vi "Main.vi"() -> ()   [LabVIEW 2020]
uses:
  Definitions/Test States.ctl
  Definitions/State Types.ctl
  lv_src/Nominal Client/Nominal Client.lvclass
  lv_src/datasources/dataset/dataset.lvclass
  lv_src/Run/Run.lvclass
  lv_src/Nominal Client/Nominal Client.lvclass/Nominal Client.ctl
  48055549-f21b-4638-95ef-231369349838.vi
  <vilib>/Analysis/1siggen.llb/Ramp Pattern by Samples.vi
  <vilib>/DAQmx/write.llb/DAQmx Write (Analog DBL 1Chan 1Samp).vi
  dc8b2421-dc48-4948-9209-d90b052b0a2b.vi
  <extravilib>/ChannelInstances/Tag-bool/Write With Abort.vi
  lv_src/Nominal Client/private_data.set.vi
  <vilib>/Utility/file.llb/Application Directory.vi
  <vilib>/Utility/error.llb/Error Cluster From Error Code.vi
  submodules/reqwest-labview/lv-src/reqwest/create.vi
  lv_src/Nominal Client/Palette Items/who_am_i.vi
  lv_src/Nominal Client/asset.get.vi
  <vilib>/DAQmx/miscellaneous.llb/DAQmx Fill In Error Info.vi
  <extravilib>/ChannelInstances/Tag-bool/Instantiate.vi
  <extravilib>/ChannelInstances/Tag-bool/Endpoint.vi
  lv_src/User/User.lvclass
  lv_src/nominal types/workspace/workspace.lvclass
  submodules/reqwest-labview/lv-src/reqwest/reqwest.lvclass
  <vilib>/Analysis/NI_AALBase.lvlib
  lv_src/event/event.lvclass
  lv_src/asset/asset.lvclass
  submodules/nominal-streaming-labview-ffi/lv_src/Stream/Stream.lvclass
  <extravilib>/ChannelInstances/Tag-bool.lvlib
panel:
  out "Status":string
  out "Acceleration":waveform(dbl)[](graph)=[{"t0"=timestamp(3854950321.550671 s since 1904-01-01), "dt"=1.9999999999999998e-05, "Y"=array[50000 elements], "attributes"=variant("NI_ChannelName"=variant(string "Accelerometers/ai0"), "NI_UnitDescription"=variant(string "Volts"))}, {"t0"=timestamp(3854950321.550671 s since 1904-01-01), "dt"=1.9999999999999998e-05, "Y"=array[50000 elements], "attributes"=variant("NI_ChannelName"=variant(string "Accelerometers/ai1"), "NI_UnitDescription"=variant(string "Volts"))}, {"t0"=timestamp(3854950321.550671 s since 1904-01-01), "dt"=1.9999999999999998e-05, "Y"=array[50000 elements], "attributes"=variant("NI_ChannelName"=variant(string "VoltageInput/ai2"), "NI_UnitDescription"=variant(string "Volts"))}]
  out "Fan Speed":dbl[](graph)=[2691.1676625669315]
  out "Temperature":dbl(slide) scale=15.0..35.0
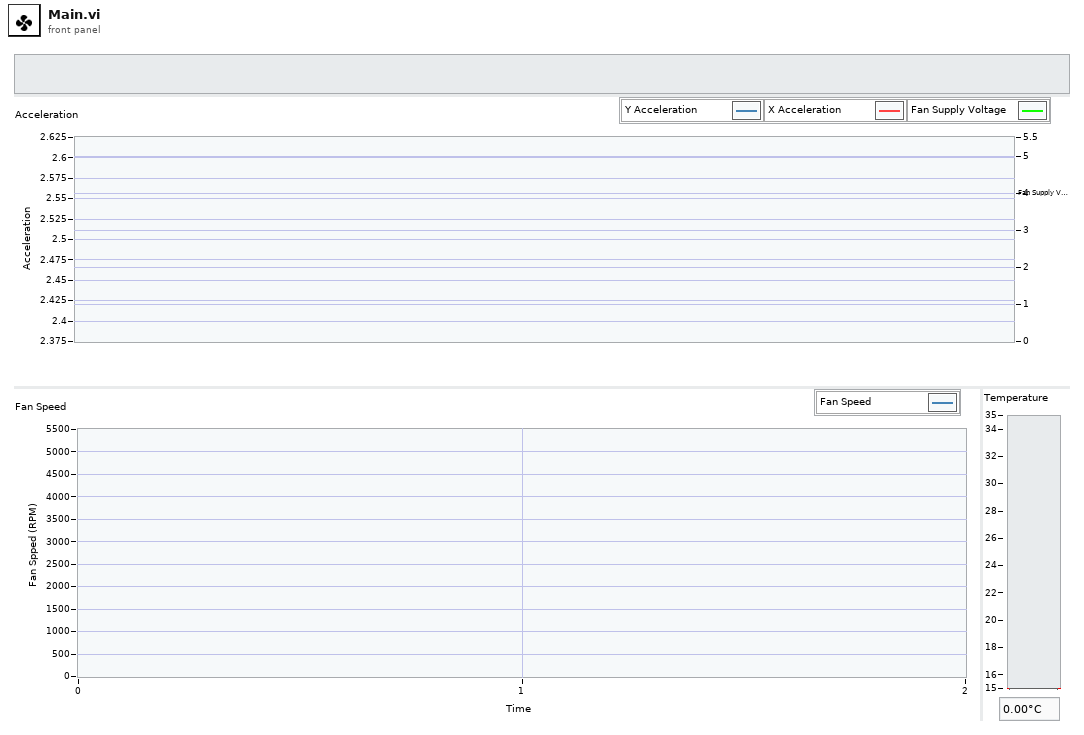
[diagram p1: front panel]
types:
  T1 = typedef "State Types.ctl" = cluster{"Nominal Client":refnum<class "Nominal Client.lvclass">, "dataset":refnum<class "dataset.lvclass">, "Run":refnum<class "Run.lvclass">, "Test Levels":dbl[], "Current Test Level":dbl, "DAQmx Task":refnum<k21>}
  T2 = typedef "Test States.ctl" = enum16{"Configuring Test Levels", "Setting Fan Voltage", "Fan Settling", "Test in Progress", "Setting Safe State", "Cooling Down"}
  T3 = typedef "Tag-bool.lvlib/))Channel.ctl" = refnum<queue>
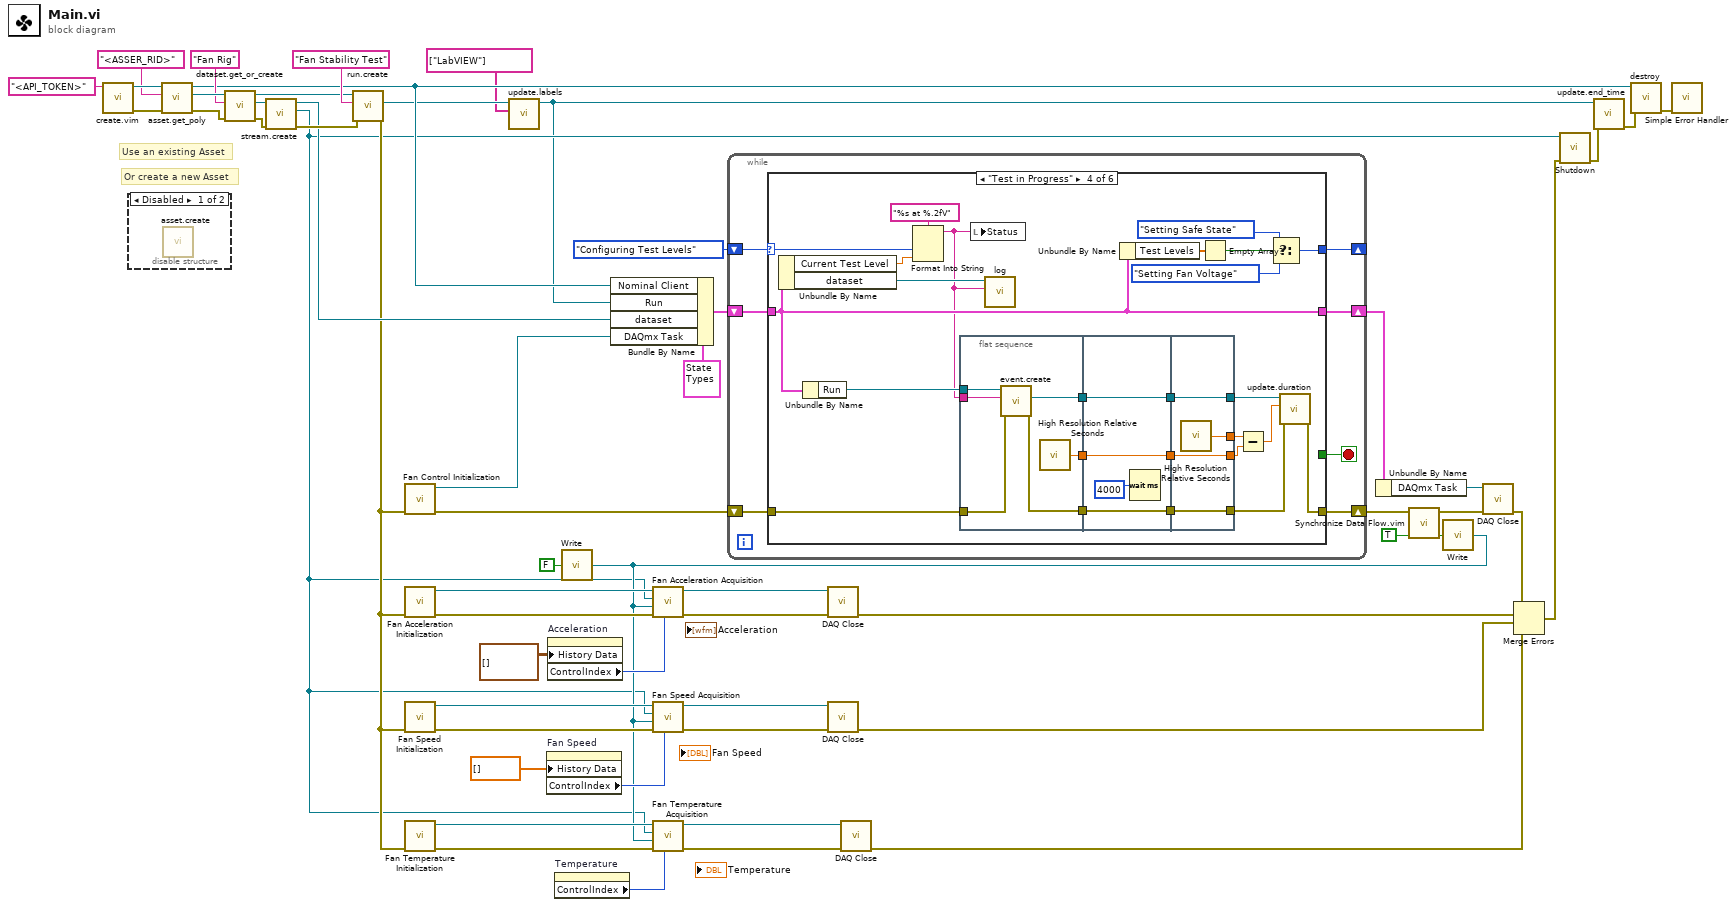
[diagram p0: block diagram]
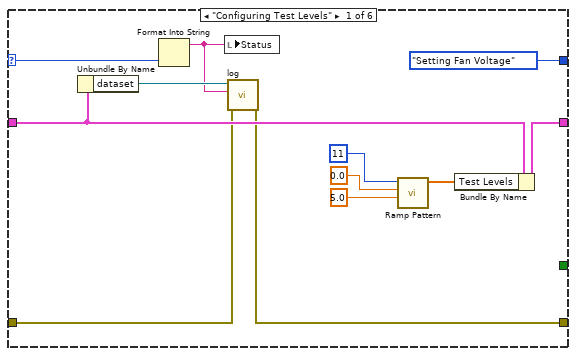
[diagram p3: hidden frame]
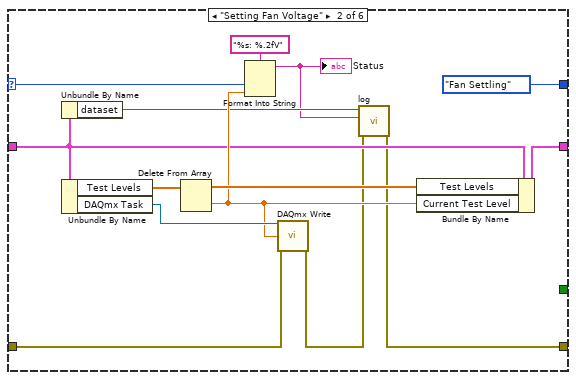
[diagram p4: hidden frame]
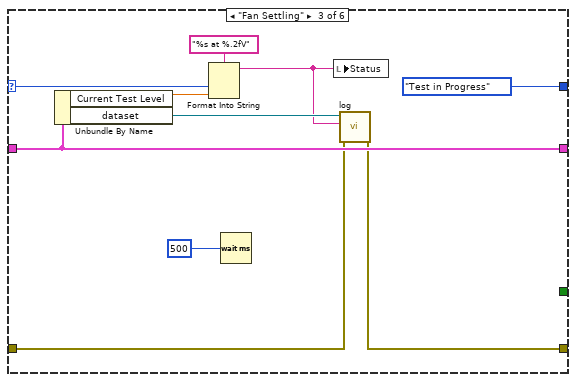
[diagram p5: hidden frame]
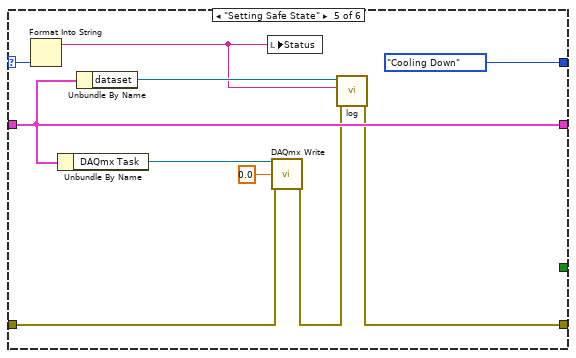
[diagram p6: hidden frame]
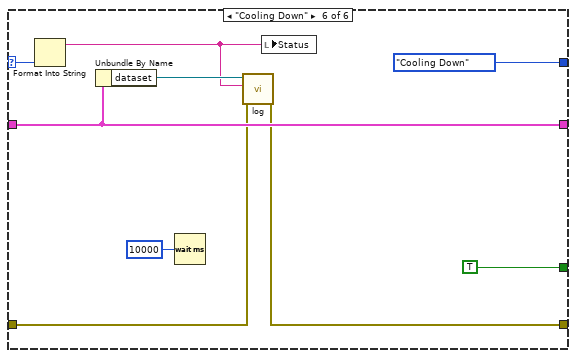
[diagram p7: hidden frame]
diagram:
  # "Or create a new Asset"
  # "Use an existing Asset"
  n1 = call "create.vim"("API Token (string or path)"="<API_TOKEN>") -> ("error out"=w55:errorcluster, "Nominal Client"=w57:refnum<class "Nominal Client.lvclass">)  [unwired: 8 in, 1 out]
  n2 = disable-structure shown="Disabled" {
    frame Disabled {
      n3 = call "asset.create.vi"() -> ()  [unwired: 9 in, 3 out]
    }
    frame Enabled {
    }
  }
  n4 = call-poly "asset.get_poly.vi"("error in"=w55, "Asset RID"="<ASSER_RID>", "Nominal Client in"=w57) -> ("error out"=w46:errorcluster, "Asset"=w52:refnum<class "asset.lvclass">, "Nominal Client out"=w39:refnum<class "Nominal Client.lvclass">)  [unwired: 6 in]
  n5 = call "dataset.get_or_create.vi"("error in"=w46, "Datascope Name"="Fan Rig", "asset in"=w52) -> ("error out"=w45:errorcluster, "dataset"=w50:refnum<class "dataset.lvclass">, "asset out"=w47:refnum<class "asset.lvclass">)  [unwired: 6 in]
  n6 = call "stream.create.vi"("error in (no error)"=w45, "dataset in"=w50) -> ("error out"=w44:errorcluster, "Stream"=w6:refnum<class "Stream.lvclass">, "dataset out"=w38:refnum<class "dataset.lvclass">)  [unwired: 7 in]
  n7 = call "run.create.vi"("error in"=w44, "Title"="Fan Stability Test", "asset in"=w47) -> ("error out"=w8:errorcluster, "Run"=w3:refnum<class "Run.lvclass">)  [unwired: 6 in, 1 out]
  n8 = call "Fan Control Initialization.vi"("error in"=w8) -> ("error out"=w13:errorcluster, "DAQmx Task"=w14:refnum<k21>)  [unwired: 9 in]
  n9 = call "Fan Acceleration Initialization.vi"("error in"=w8) -> ("error out"=w26:errorcluster, "DAQmx Task"=w27:refnum<k21>)  [unwired: 9 in]
  n10 = call "Fan Speed Initialization.vi"("error in"=w8) -> ("error out"=w24:errorcluster, "DAQmx Task Out"=w25:refnum<k21>)  [unwired: 9 in]
  n11 = call "Fan Temperature Initialization.vi"("error in"=w8) -> ("error out"=w11:errorcluster, "DAQmx Task"=w12:refnum<k21>)  [unwired: 9 in]
  n12 = call "update.labels.vi"("labels"=string[] ["LabVIEW"], "Run in"=w3) -> ("Run out"=w2:refnum<class "Run.lvclass">)  [unwired: 8 in, 1 out]
  n13 = property on="Fan Speed" class="WFChart (strict)"("History Data"=dbl[] []) -> ("ControlIndex"=w28:i32)  [unwired: 2 in, 2 out]
  n14 = property on="Acceleration" class="WFChart (strict)"("History Data"=waveform(dbl)[][] []) -> ("ControlIndex"=w29:i32)  [unwired: 2 in, 2 out]
  n15 = property on="Temperature" class="Slide (strict)"() -> ("ControlIndex"=w5:i32)  [unwired: 2 in, 2 out]
  n16 = call <extravilib>:"Write.vi"("element"=FALSE ("stop")) -> ("channel"=w7:T3)  [unwired: 1 out]
  n17 = Bundle By Name(cluster=T1 {"Nominal Client"=refnum, "dataset"=refnum, "Run"=refnum, "Test Levels"=[], "Current Test Level"=0.0, "DAQmx Task"=""} ("State Type"), "Nominal Client"=w39, "Run"=w2, "dataset"=w38, "DAQmx Task"=w14) -> (w37:T1)
  n18 = call "Fan Acceleration Acquisition.vi"("Acceleration Control Index"=w29, "error in"=w26, "stop"=w7, "Stream"=w6, "DAQmx Task In"=w27) -> ("error out"=w19:errorcluster, "DAQmx Task Out"=w20:refnum<k21>)  [unwired: 5 in]
  n19 = call "Fan Speed Acquisition.vi"("Control Index"=w28, "error in (no error)"=w24, "channel"=w7, "Stream in"=w6, "DAQmx Task In"=w25) -> ("error out"=w17:errorcluster, "DAQmx Task Out"=w18:refnum<k21>)  [unwired: 5 in]
  n20 = call "Fan Temperature Acquisition.vi"("Control Index"=w5, "error in (no error)"=w11, "channel"=w7, "Stream in"=w6, "DAQmx Task In"=w12) -> ("error out"=w10:errorcluster, "DAQmx Task Out"=w9:refnum<k21>)  [unwired: 5 in]
  n21 = while {
    shift-right: [w63] -> _
    shift-left: Test_States."Configuring Test Levels" ("states") -> [w64]
    shift-right: [w60] -> w35
    shift-left: w13 -> [w61]
    shift-right: [w58] -> w36
    shift-left: w37 -> [w59]
    stop <- w62 stop-if-true
    n22 = case shown="\"Test in Progress\"" w64 {
      selector: w64 -> [w72 w87 w98 w107 w146 w155]
      tunnel: [Test_States."Setting Fan Voltage" ("states") Test_States."Fan Settling" ("states") Test_States."Test in Progress" ("states") w122 Test_States."Cooling Down" ("states") Test_States."Cooling Down" ("states")] -> w63
      tunnel: [_ _ _ _ _ TRUE] -> w62
      tunnel: w61 -> [w66 w89 w93 w121 w147 w151]
      tunnel: [w65 w77 w92 w110 w140 w150] -> w60
      tunnel: w59 -> [w69 w81 w96 w104 w144 w154]
      tunnel: [w71 w85 w96 w104 w144 w154] -> w58
      frame "Configuring Test Levels" {
        n23 = Unbundle By Name(w69) -> ("dataset"=w68:refnum<class "dataset.lvclass">)
        n24 = Format Into String(w72) -> (resulting string=w67:string)  [unwired: 3 in, 1 out]
        n25 = local write "Status"(w67) -> ()
        n26 = call "log.vi"("error in (no error)"=w66, "Message"=w67, "dataset in"=w68) -> ("error out"=w65:errorcluster)  [unwired: 7 in, 1 out]
        n27 = call-poly <vilib>:"Ramp Pattern.vi"("start"=5.0 ("end"), "end"=0.0 ("start"), "samples"=11) -> ("Ramp Pattern"=w70:dbl[])  [unwired: 7 in, 1 out]
        n28 = Bundle By Name(cluster=w69, "Test Levels"=w70) -> (w71:T1)
      }
      frame "Setting Fan Voltage" {
        n29 = Unbundle By Name(w81) -> ("dataset"=w80:refnum<class "dataset.lvclass">)
        n30 = Unbundle By Name(w81) -> ("Test Levels"=w86:dbl[], "DAQmx Task"=w83:refnum<k21>)
        n31 = Delete From Array(array=w86) -> (deleted portion=w82:dbl, array with subset deleted=w84:dbl[])  [unwired: 2 in]
        n32 = Format Into String(format string="%s: %.2fV", w87, w82) -> (resulting string=w79:string)  [unwired: 2 in, 1 out]
        "Status" <- w79
        n33 = call-poly <vilib>:"DAQmx Write.vi"("task/channels in"=w83, "data"=w82, "error in"=w89) -> ("error out"=w78:errorcluster)  [unwired: 10 in, 2 out]
        n34 = call "log.vi"("error in (no error)"=w78, "Message"=w79, "dataset in"=w80) -> ("error out"=w77:errorcluster)  [unwired: 7 in, 1 out]
        n35 = Bundle By Name(cluster=w81, "Test Levels"=w84, "Current Test Level"=w82) -> (w85:T1)
      }
      frame "Fan Settling" {
        n36 = Unbundle By Name(w96) -> ("Current Test Level"=w95:dbl, "dataset"=w94:refnum<class "dataset.lvclass">)
        n37 = Format Into String(format string="%s at %.2fV", w98, w95) -> (resulting string=w91:string)  [unwired: 2 in, 1 out]
        n38 = Wait (ms)(milliseconds to wait=u32 500) -> ()  [unwired: 1 out]
        n39 = local write "Status"(w91) -> ()
        n40 = call "log.vi"("error in (no error)"=w93, "Message"=w91, "dataset in"=w94) -> ("error out"=w92:errorcluster)  [unwired: 7 in, 1 out]
      }
      frame "Test in Progress" {
        n41 = Unbundle By Name(w104) -> ("Current Test Level"=w106:dbl, "dataset"=w102:refnum<class "dataset.lvclass">)
        n42 = Unbundle By Name(w104) -> ("Run"=w105:refnum<class "Run.lvclass">)
        n43 = Format Into String(format string="%s at %.2fV", w107, w106) -> (resulting string=w101:string)  [unwired: 2 in, 1 out]
        n44 = flat-sequence {
          tunnel: w121 -> [w131]
          tunnel: [w130] -> w117
          tunnel: [w129] -> w113
          tunnel: [w128] -> w112
          tunnel: w105 -> [w127]
          tunnel: w101 -> [w126]
          tunnel: [w134] -> w118
          tunnel: w117 -> [w134]
          tunnel: [w133] -> w114
          tunnel: w113 -> [w133]
          tunnel: w112 -> [w132]
          tunnel: [w132] -> w111
          tunnel: [w139] -> w120
          tunnel: [w138] -> w119
          tunnel: w118 -> [w138]
          tunnel: [w137] -> w115
          tunnel: w114 -> [w137]
          tunnel: w111 -> [w136]
          tunnel: [w136] -> w109
          frame #0 {
            n45 = call "event.create.vi"("error in (no error)"=w131, "Name"=w126, "Run in"=w127) -> ("error out"=w128:errorcluster, "event"=w129:refnum<class "event.lvclass">)  [unwired: 6 in, 1 out]
            n46 = call <vilib>:"High Resolution Relative Seconds.vi"() -> ("relative seconds"=w130:dbl)
          }
          frame #1 {
            n47 = Wait (ms)(milliseconds to wait=u32 4000) -> ()  [unwired: 1 out]
          }
          frame #2 {
            n48 = call <vilib>:"High Resolution Relative Seconds.vi"() -> ("relative seconds"=w139:dbl)
          }
        }
        n49 = local write "Status"(w101) -> ()
        n50 = call "log.vi"("Message"=w101, "dataset in"=w102) -> ()  [unwired: 8 in, 2 out]
        n51 = Unbundle By Name(w104) -> ("Test Levels"=w103:dbl[])
        n52 = Empty Array?(array=w103) -> (empty?=w125:bool)
        n53 = Subtract(x=w120, y=w119) -> (x-y=w116:dbl)
        n54 = Select(t=Test_States."Setting Safe State" ("states"), s=w125, f=Test_States."Setting Fan Voltage" ("states")) -> (s? t:f=w122:T2)
        n55 = call "update.duration.vi"("error in (no error)"=w109, "Duration (s)"=w116, "event in"=w115) -> ("error out"=w110:errorcluster)  [unwired: 7 in, 1 out]
      }
      frame "Setting Safe State" {
        n56 = Format Into String(w146) -> (resulting string=w142:string)  [unwired: 3 in, 1 out]
        n57 = Unbundle By Name(w144) -> ("DAQmx Task"=w145:refnum<k21>)
        n58 = Unbundle By Name(w144) -> ("dataset"=w143:refnum<class "dataset.lvclass">)
        n59 = local write "Status"(w142) -> ()
        n60 = call-poly <vilib>:"DAQmx Write.vi"("task/channels in"=w145, "data"=0.0, "error in"=w147) -> ("error out"=w141:errorcluster)  [unwired: 10 in, 2 out]
        n61 = call "log.vi"("error in (no error)"=w141, "Message"=w142, "dataset in"=w143) -> ("error out"=w140:errorcluster)  [unwired: 7 in, 1 out]
      }
      frame "Cooling Down" {
        n62 = Format Into String(w155) -> (resulting string=w152:string)  [unwired: 3 in, 1 out]
        n63 = Unbundle By Name(w154) -> ("dataset"=w153:refnum<class "dataset.lvclass">)
        n64 = Wait (ms)(milliseconds to wait=u32 10000) -> ()  [unwired: 1 out]
        n65 = call "log.vi"("error in (no error)"=w151, "Message"=w152, "dataset in"=w153) -> ("error out"=w150:errorcluster)  [unwired: 7 in, 1 out]
        n66 = local write "Status"(w152) -> ()
      }
    }
  }
  n67 = call "DAQ Close.vi"("error in"=w19, "DAQmx Task In"=w20) -> ("error out"=w16:errorcluster)  [unwired: 9 in]
  n68 = call "DAQ Close.vi"("error in"=w17, "DAQmx Task In"=w18) -> ("error out"=w15:errorcluster)  [unwired: 9 in]
  n69 = call "DAQ Close.vi"("error in"=w10, "DAQmx Task In"=w9) -> ("error out"=w4:errorcluster)  [unwired: 9 in]
  n70 = Unbundle By Name(w36) -> ("DAQmx Task"=w23:refnum<k21>)
  n71 = call "Synchronize Data Flow.vim"("input 4"=TRUE ("element"), "input 1"=w35) -> ("output 4"=w33:bool, "output 1"=w22:errorcluster)  [unwired: 2 in, 2 out]
  n72 = call <extravilib>:"Write.vi"("element"=w33, "channel"=w7) -> ()  [unwired: 1 out]
  n73 = call "DAQ Close.vi"("error in"=w22, "DAQmx Task In"=w23) -> ("error out"=w21:errorcluster)  [unwired: 9 in]
  n74 = Merge Errors(w21, w16, w15, w4) -> (w48:errorcluster)
  n75 = call "Shutdown.vi"("error in (no error)"=w48, "Nominal Streaming in"=w6) -> ("error out"=w43:errorcluster)  [unwired: 8 in, 1 out]
  n76 = call "update.end_time.vi"("error in (no error)"=w43, "Run in"=w2) -> ("error out"=w42:errorcluster)  [unwired: 8 in, 1 out]
  n77 = call "destroy.vi"("error in"=w42, "Nominal Client"=w39) -> ("error out"=w54:errorcluster)  [unwired: 9 in]
  n78 = call <vilib>:"Simple Error Handler.vi"("error in (no error)"=w54) -> ()  [unwired: 4 in, 5 out]
